vi "wireUnbundle.vi"(0 "vi reference":refnum<vi>, 2 "UnbundleByNameReference":refnum<vi>, 3 "error in":errorcluster, 4 "Controls":cluster{"Style":u32, "Label.Text":string, i32}[](array[cluster]), 8 "NofInputs":i32) -> (9 "error out":errorcluster)   [LabVIEW 2009, in "HGF_VisitorGenerator.lvlib"]
doc: "wire unbundle by name node in visitors action.vi"
uses:
  HGF_VisitorGenerator.lvlib
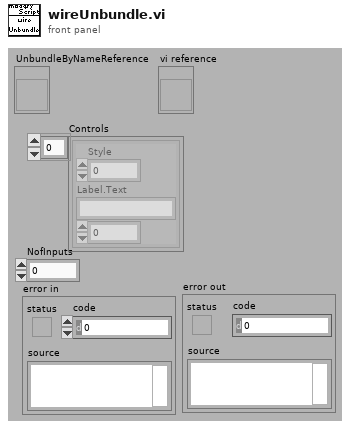
[diagram p1: front panel]
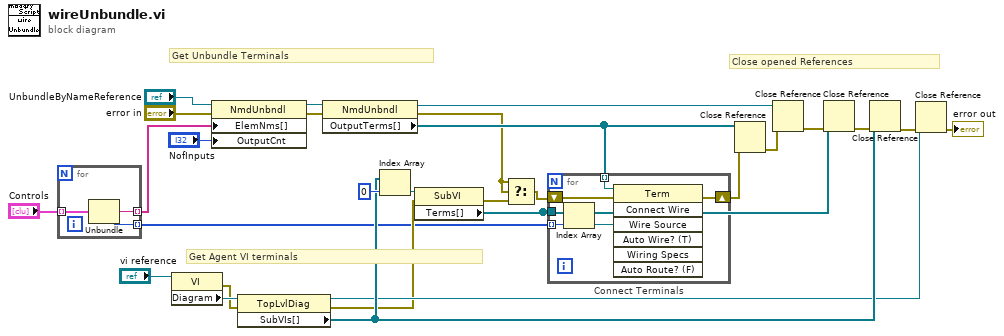
[diagram p0: block diagram]
diagram:
  # "Close opened References"
  # "Get Unbundle Terminals"
  # "Get Agent VI terminals"
  n1 = for {
    tunnel: "Controls" -> [w31] mode=indexing
    tunnel: [w30] -> w15 mode=indexing
    tunnel: [w29] -> w6 mode=indexing
    n2 = Unbundle(w31) -> ("Label.Text"=w30:string, w29:i32)  [unwired: 1 out]
  }
  n3 = property class="VI"(reference="vi reference") -> (error out=w9:errorcluster, "Diagram"=w23:refnum<vi>)  [unwired: 1 in, 1 out]
  n4 = property class="NmdUnbndl"(reference="UnbundleByNameReference", error in="error in", "ElemNms[]"=w15, "OutputCnt"="NofInputs") -> (reference out=w18:refnum<vi>, error out=w20:errorcluster)
  n5 = property class="TopLvlDiag"(reference=w23, error in=w9) -> (reference out=w24:refnum<vi>, error out=w8:errorcluster, "SubVIs[]"=w27:refnum<vi>[])
  n6 = property class="NmdUnbndl"(reference=w18, error in=w20) -> (reference out=w19:refnum<vi>, error out=w2:errorcluster, "OutputTerms[]"=w5:refnum<vi>[])
  n7 = Index Array(array=w27, index=0) -> (element=w12:refnum<vi>)
  n8 = property class="SubVI"(reference=w12, error in=w8) -> (error out=w3:errorcluster, "Terms[]"=w7:refnum<vi>[])  [unwired: 1 out]
  n9 = Select(t=w2, s=w2, f=w3) -> (s? t:f=w1:errorcluster)
  n10 = for "Connect Terminals" {
    tunnel: w7 -> [w37]
    tunnel: w6 -> [w36] mode=indexing
    tunnel: w5 -> [w35] mode=indexing
    shift-right: [w32] -> w4
    shift-left: w1 -> [w33]
    n11 = Index Array(array=w37, index=w36) -> (element=w34:refnum<vi>)
    n12 = invoke class="Term" method="Connect Wire"(reference=w35, error in=w33, "Wire Source"=w34) -> (error out=w32:errorcluster)  [unwired: 4 in, 6 out]
  }
  n13 = Close Reference(reference=w5, error in (no error)=w4) -> (error out=w21:errorcluster)
  n14 = Close Reference(reference=w19, error in (no error)=w21) -> (error out=w11:errorcluster)
  n15 = Close Reference(reference=w7, error in (no error)=w11) -> (error out=w10:errorcluster)
  n16 = Close Reference(reference=w27, error in (no error)=w10) -> (error out=w26:errorcluster)
  n17 = Close Reference(reference=w24, error in (no error)=w26) -> (error out=→"error out":errorcluster)
